vi "Init Device.vi"(8 "error in (no error)":errorcluster, 10 "Settings":T1={"Simulation"=enum."off", "Timeout"={"Value"=100.0, "Min"=100.0, "Max"=5000.0, "StepSize"=100.0, "Tolerance"=0.0, "valueactual"=0.0}, "Save"=enum."off", "LocalSavingPath"=path "c:/temp", "MeasurementMode"={"Channel0"=enum."Energy", "Channel1"=enum."Energy", "Channel2"=enum."Energy", "Channel3"=enum."Energy"}, "ExternalTrigger"={"Channel0"=enum."off", "Channel1"=enum."off", "Channel2"=enum."off", "Channel3"=enum."off"}, "Wavelength"={"Channel0"=enum."248", "Channel1"=enum."248", "Channel2"=enum."248", "Channel3"=enum."248"}, "PulseWidth"={"Channel0"=enum."50uS", "Channel1"=enum."50uS", "Channel2"=enum."50uS", "Channel3"=enum."50uS"}, "EnergyRange"={"Channel0"=enum."20.00J", "Channel1"=enum."20.00J", "Channel2"=enum."20.00J", "Channel3"=enum."20.00J"}, "EnableCh"={"Channel0"=enum."Enable", "Channel1"=enum."Enable", "Channel2"=enum."Enable", "Channel3"=enum."Enable"}, "NumberOfCh"={"Value"=0.0, "Min"=0.0, "Max"=10.0, "StepSize"=1.0, "Tolerance"=0.0, "valueactual"=0.0}}, 11 "Ophir Pulsar in":refnum<class "Ophir Pulsar.lvclass">) -> (0 "error out":errorcluster, 2 "Serial Number":string, 3 "Ophir Pulsar out":refnum<class "Ophir Pulsar.lvclass">)   [LabVIEW 2013, in "Ophir Pulsar.lvclass"]
uses:
  Ophir Pulsar.lvclass
  settings_TypDef.ctl
  OnOffTypeDef.ctl
  Measurement_Mode.ctl
  External_Trigger.ctl
  Wavelength.ctl
  Pulse_Width.ctl
  Energy_Range.ctl
  Enable_Disable Channel.ctl
  Ophir Pulsar.lvclass/Ophir Pulsar.ctl
panel:
  out "serialNumber":string
  out "hDevice":i32
  out "deviceName":string
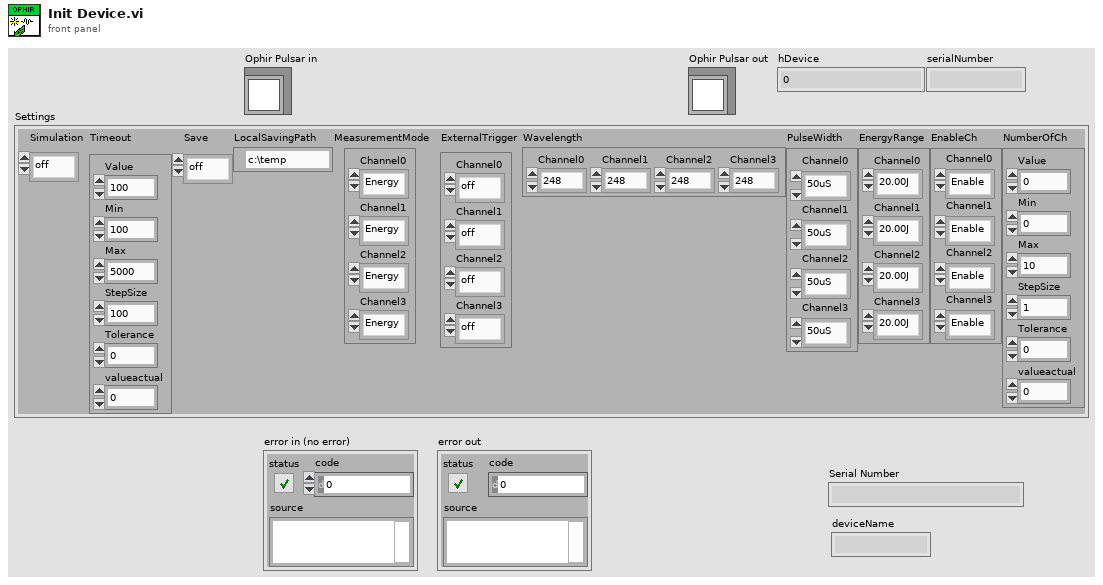
[diagram p1: front panel]
types:
  T1 = typedef "Ophir Pulsar.lvclass/settings_TypDef.ctl" = cluster{"Simulation":T2, "Timeout":cluster{"Value":dbl, "Min":dbl, "Max":dbl, "StepSize":dbl, "Tolerance":dbl, "valueactual":dbl}, "Save":T2, "LocalSavingPath":path, "MeasurementMode":cluster{"Channel0":T3, "Channel1":enum16{"Energy", "Power"}, "Channel2":enum16{"Energy", "Power"}, "Channel3":enum16{"Energy", "Power"}}, "ExternalTrigger":cluster{"Channel0":T4, "Channel1":enum16{"off", "on"}, "Channel2":enum16{"off", "on"}, "Channel3":enum16{"off", "on"}}, "Wavelength":cluster{"Channel0":T5, "Channel1":T5, "Channel2":T5, "Channel3":T5}, "PulseWidth":cluster{"Channel0":T6, "Channel1":T6, "Channel2":T6, "Channel3":T6}, "EnergyRange":cluster{"Channel0":T7, "Channel1":T7, "Channel2":T7, "Channel3":T7}, "EnableCh":cluster{"Channel0":T8, "Channel1":T8, "Channel2":T8, "Channel3":T8}, "NumberOfCh":cluster{"Value":dbl, "Min":dbl, "Max":dbl, "StepSize":dbl, "Tolerance":dbl, "valueactual":dbl}}
  T2 = typedef "OnOffTypeDef.ctl" = enum16{"off", "on"}
  T3 = typedef "Ophir Pulsar.lvclass/Measurement_Mode.ctl" = enum16{"Power", "Energy"}
  T4 = typedef "Ophir Pulsar.lvclass/External_Trigger.ctl" = enum16{"off", "on"}
  T5 = typedef "Ophir Pulsar.lvclass/Wavelength.ctl" = enum16{"248", "355", "532", "800", "2940", "193"}
  T6 = typedef "Ophir Pulsar.lvclass/Pulse_Width.ctl" = enum16{"50uS", "1.0mS"}
  T7 = typedef "Ophir Pulsar.lvclass/Energy_Range.ctl" = enum16{"20.00J", "4.00J", "400mJ", "40.0mJ", "4.00mJ"}
  T8 = typedef "Ophir Pulsar.lvclass/Enable_Disable Channel.ctl" = enum16{"Enable", "Disable"}
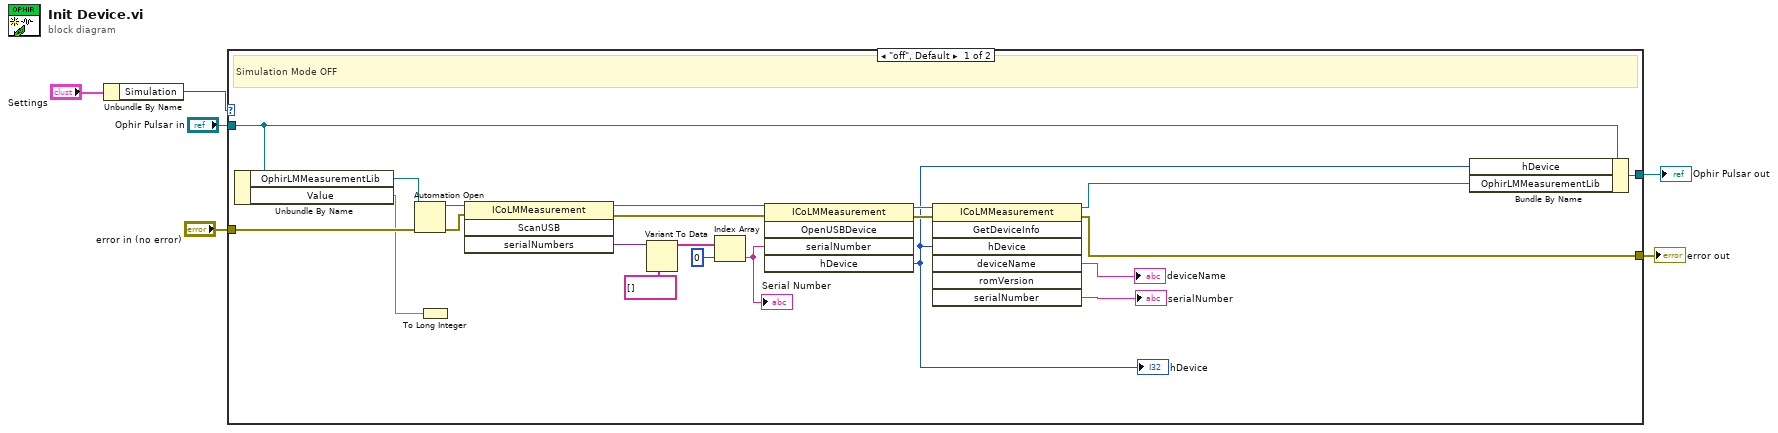
[diagram p0: block diagram]
diagram:
  n1 = Unbundle By Name("Settings") -> ("Simulation"=w5:T2)
  n2 = case shown="\"off\", Default" w5 {
    tunnel: "error in (no error)" -> [w25 w28]
    tunnel: [w9 w28] -> w3
    tunnel: "Ophir Pulsar in" -> [w19 w29]
    tunnel: [w18 w29] -> w4
    frame "off", Default {
      # "Simulation Mode OFF"
      n3 = Unbundle By Name(w19) -> ("OphirLMMeasurementLib"=w26:refnum<k7>, "Value"=w10:dbl)
      n4 = Automation Open(error in (no error)=w25, Automation Refnum=w26) -> (Automation Refnum=w27:refnum<k7>, error out=w20:errorcluster)  [unwired: 2 in]
      n5 = To Long Integer(number=w10) -> ()  [unwired: 1 out]
      n6 = invoke class="ICoLMMeasurement" method="ScanUSB"(reference=w27, error in=w20) -> (reference out=w14:refnum<k7>, error out=w16:errorcluster, "serialNumbers"=w21:variant)  [unwired: 2 in, 1 out]
      n7 = Variant To Data(type=string[] [], Variant=w21) -> (data=w24:string[])  [unwired: 1 in, 1 out]
      n8 = Index Array(array=w24, index=0) -> (element=w17:string)
      "Serial Number" <- w17
      n9 = invoke class="ICoLMMeasurement" method="OpenUSBDevice"(reference=w14, error in=w16, "serialNumber"=w17) -> (reference out=w13:refnum<k7>, error out=w15:errorcluster, "hDevice"=w11:i32)  [unwired: 2 in, 2 out]
      "hDevice" <- w11
      n10 = invoke class="ICoLMMeasurement" method="GetDeviceInfo"(reference=w13, error in=w15, "hDevice"=w11) -> (reference out=w12:refnum<k7>, error out=w9:errorcluster, "deviceName"=→"deviceName":string, "serialNumber"=→"serialNumber":string)  [unwired: 4 in, 3 out]
      n11 = Bundle By Name(cluster=w19, "hDevice"=w11, "OphirLMMeasurementLib"=w12) -> (w18:refnum<class "Ophir Pulsar.lvclass">)
    }
    frame "on" {
      # "Simulation Mode ON"
    }
  }
  "Ophir Pulsar out" <- w4
  "error out" <- w3
